vi "날시.vi"() -> ()   [LabVIEW 2014]
panel:
  out "날시":string
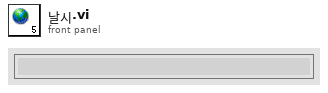
[diagram p1: front panel]
diagram:
